vi "Getmsg_1.vi"(8 "error in (no error)":errorcluster, 11 "OneOfTemplate in":refnum<class "w4lvgrpc_ToClient_payload.lvclass">) -> (0 "error out":errorcluster, 2 "Get_Val":T1, 3 "OneOfTemplate out":refnum<class "w4lvgrpc_ToClient_payload.lvclass">)   [LabVIEW 2019, in "Generated_client.lvlib" / "w4lvgrpc_ToClient_payload.lvclass"]
uses:
  w4lvgrpc_ToClient_payload.lvclass
  w4lvgrpc_Msg_ToClient_1.ctl
  Generated_client.lvlib
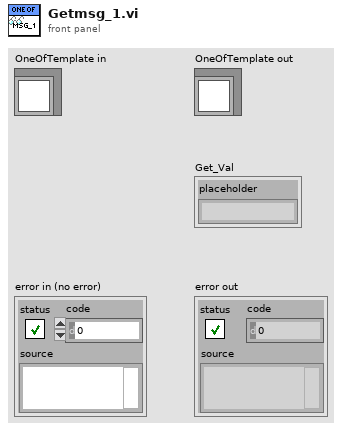
[diagram p1: front panel]
types:
  T1 = typedef "Generated_client.lvlib/w4lvgrpc_Msg_ToClient_1.ctl" = cluster{"placeholder":string}
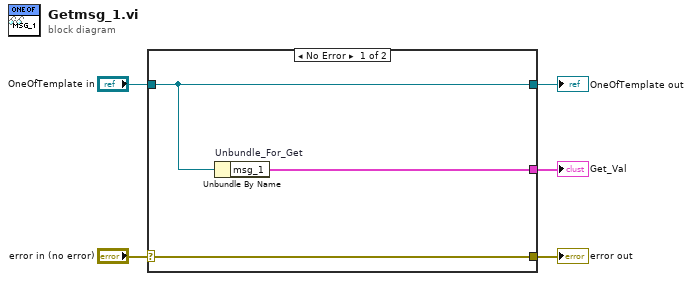
[diagram p0: block diagram]
diagram:
  n1 = case shown="No Error" "error in (no error)" {
    selector: "error in (no error)" -> [w8 w9]
    tunnel: [w8 w9] -> w4
    tunnel: [w7 w10] -> w2
    tunnel: "OneOfTemplate in" -> [w7 w10]
    tunnel: [w6 _] -> w1
    frame No Error {
      n2 = Unbundle By Name "Unbundle_For_Get"(w7) -> ("msg_1"=w6:T1)
    }
    frame Error {
    }
  }
  "error out" <- w4
  "OneOfTemplate out" <- w2
  "Get_Val" <- w1
